vi "Read menu item.vi"(8 "Error In":errorcluster, 11 "RunTimeMenu":refnum<k24>[](array[refnum])) -> (0 "Error Out":errorcluster, 2 "Run Time Menu":T1[](array[typedef]))   [LabVIEW 2015, in "Configuration Tool.lvlib"]
uses:
  Configuration Tool.lvlib
  NationalInstruments.VeriStand.XMLReader
  XML Controls/Menu Item.ctl
  XML Controls/Execution Types.ctl
  XML Controls/Path Cluster.ctl
  XML Controls/Dependency three item small.ctl
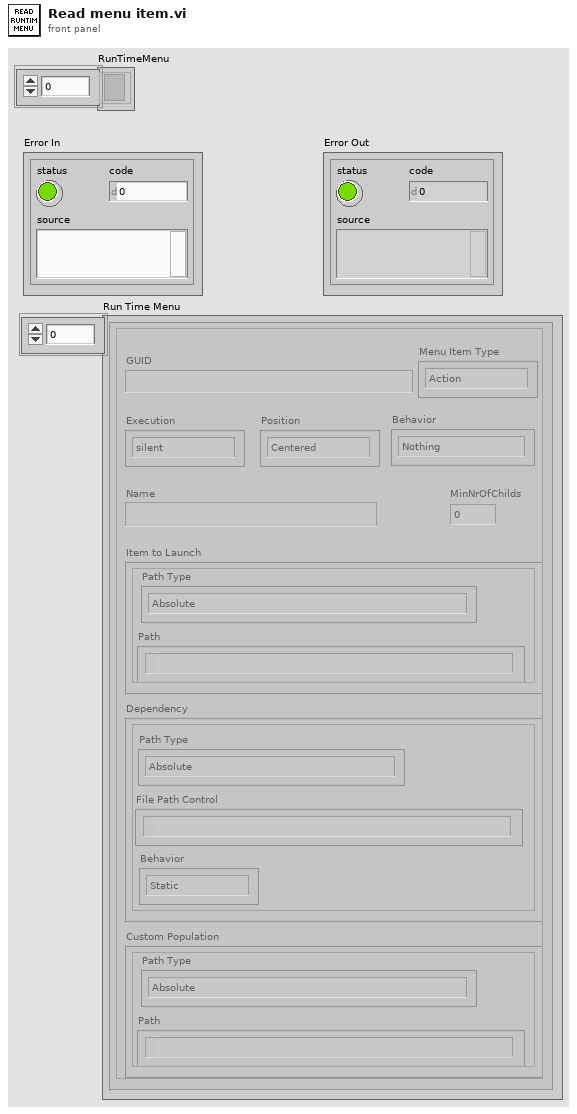
[diagram p1: front panel]
types:
  T1 = typedef "Configuration Tool.lvlib/Menu Item.ctl" = cluster{"GUID":string, "Execution":T2, "MinNrOfChilds":u32, "Name":string, "Item to Launch":T3, "Dependency":T4, "Custom Population":T3, "Menu Item Type":enum16{"Action", "VI", "Separator", "Custom"}, "Behavior":enum16{"Nothing", "Open Front Panel"}, "Position":enum16{"Centered", "Mouse Pointer"}}
  T2 = typedef "Configuration Tool.lvlib/Execution Types.ctl" = enum16{"silent", "modal", "floating", "default"}
  T3 = typedef "Configuration Tool.lvlib/Path Cluster.ctl" = cluster{"Path":path, "Path Type":enum16{"Absolute", "To Base", "To Common Doc Dir", "To Application Data Dir"}}
  T4 = typedef "Configuration Tool.lvlib/Dependency three item small.ctl" = cluster{"File Path Control":path, "Path Type":enum16{"Absolute", "To Base", "To Common Doc Dir", "To Application Data Dir"}, "Behavior":enum16{"Static", "Dynamic"}}
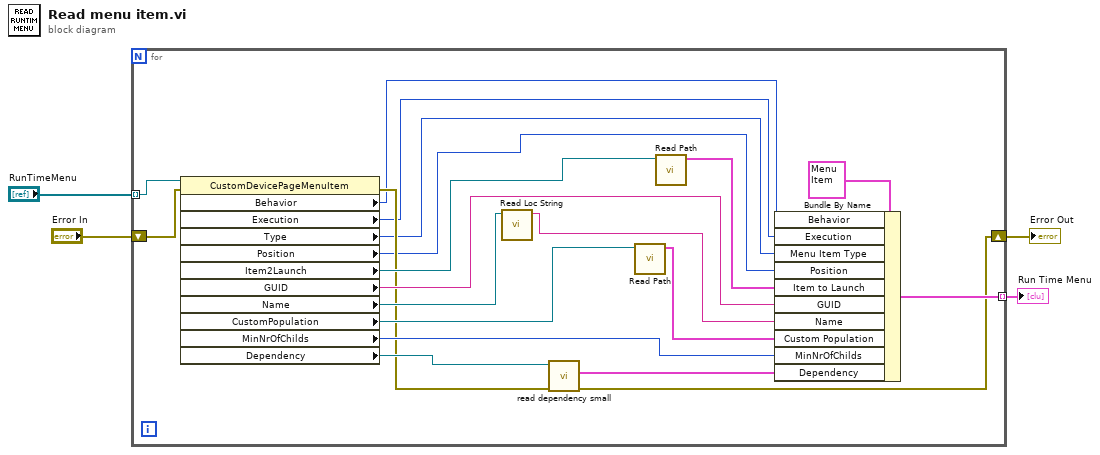
[diagram p0: block diagram]
diagram:
  n1 = for {
    tunnel: "RunTimeMenu" -> [w24] mode=indexing
    tunnel: [w16] -> w3 mode=indexing
    shift-right: [w14] -> w1
    shift-left: "Error In" -> [w15]
    n2 = property class="CustomDevicePageMenuItem"(reference=w24, error in=w15) -> (error out=w13:errorcluster, "Behavior"=w8:i32, "Execution"=w9:i32, "Type"=w10:i32, "Position"=w11:i32, "Item2Launch"=w21:refnum<k24>, "GUID"=w22:string, "Name"=w20:refnum<k24>, "CustomPopulation"=w19:refnum<k24>, "MinNrOfChilds"=w18:i32, "Dependency"=w17:refnum<k24>)  [unwired: 1 out]
    n3 = call "Read Loc String.vi"("Loc String .NET Ref"=w20) -> ("English"=w7:string)  [unwired: 8 in, 2 out]
    n4 = call "read dependency small.vi"("error in (no error)"=w13, ".NET Refnum in"=w17) -> ("error out"=w14:errorcluster, "Dependency"=w12:T4)  [unwired: 8 in]
    n5 = call "Read Path.vi"("Path .NET Ref"=w19) -> ("Path Properties"=w5:T3)  [unwired: 9 in, 1 out]
    n6 = call "Read Path.vi"("Path .NET Ref"=w21) -> ("Path Properties"=w6:T3)  [unwired: 9 in, 1 out]
    n7 = Bundle By Name(cluster=T1 {"GUID"="", "Execution"=enum."silent", "MinNrOfChilds"=0, "Name"="", "Item to Launch"={"Path"=path "", "Path Type"=enum."Absolute"}, "Dependency"={"File Path Control"=path "", "Path Type"=enum."Absolute", "Behavior"=enum."Static"}, "Custom Population"={"Path"=path "", "Path Type"=enum."Absolute"}, "Menu Item Type"=enum."Action", "Behavior"=enum."Nothing", "Position"=enum."Centered"} ("Menu Item"), "Behavior"=w8, "Execution"=w9, "Menu Item Type"=w10, "Position"=w11, "Item to Launch"=w6, "GUID"=w22, "Name"=w7, "Custom Population"=w5, "MinNrOfChilds"=w18, "Dependency"=w12) -> (w16:T1)
  }
  "Run Time Menu" <- w3
  "Error Out" <- w1
